vi "Handle Command.vi"(8 "error in":errorcluster, 10 "CMD in":refnum<class "Change Filter State CMD.lvclass">, 11 "Object In":refnum<class>) -> (0 "error out":errorcluster, 1 "Command Successful?":bool, 2 "CMD out":refnum<class "Change Filter State CMD.lvclass">, 3 "Object Out":refnum<class>)   [LabVIEW 2017, in "PAS Library.lvlib" / "Change Filter State CMD.lvclass"]
doc: "This VI will contain the code used to actually execute the request. If the request is successful, this will be indicated by the boolean output <b>Command Successful?</b>. The boolean output can then be used by the <b>Command Reply</b> which sends a reply if the reply queue is valid."
uses:
  Change Filter State CMD.lvclass
  Main/PAS.lvclass
  Change Filter State CMD.lvclass/Change Filter State CMD.ctl
  Cell/PAS Cell.lvclass/PAS Cell.ctl
  Cell/Write filter.vi
  Main/Read Cells.vi
  Main/Write Cells.vi
  Cell/PAS Cell.lvclass
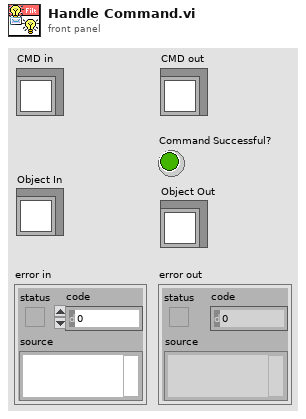
[diagram p1: front panel]
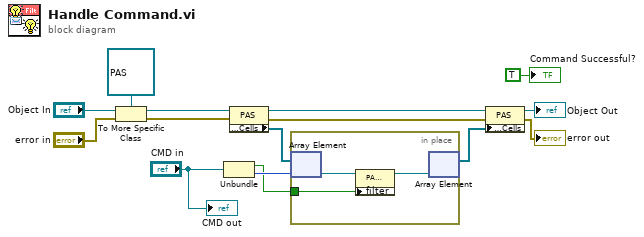
[diagram p0: block diagram]
diagram:
  n1 = To More Specific Class(target class=refnum<class "PAS.lvclass"> refnum ("PAS Library.lvlib:PAS"), reference="Object In", error in="error in") -> (specific class reference=w11:refnum<class "PAS.lvclass">, error out=w10:errorcluster)
  n2 = Unbundle("CMD in") -> (w7:bool, w8:u8)
  n3 = property class="PAS"(reference=w11, error in=w10) -> (reference out=w6:refnum<class "PAS.lvclass">, error out=w4:errorcluster, "Data Access:Cells"=w9:refnum<class "PAS Cell.lvclass">[])
  n4 = in-place {
    in-place-border: w7 -> [w17]
    n5 = in-place-array #1(w9, w8) -> (w18:refnum<class "PAS Cell.lvclass">)
    n6 = property class="PAS Cell"(reference=w18, "filter"=w17) -> (reference out=w16:refnum<class "PAS Cell.lvclass">)  [unwired: 1 in, 1 out]
    n7 = in-place-array #1(w16) -> (w5:refnum<class "PAS Cell.lvclass">[])  [unwired: 1 out]
  }
  n8 = property class="PAS"(reference=w6, error in=w4, "Data Access:Cells"=w5) -> (reference out=→"Object Out":refnum<class "PAS.lvclass">, error out=→"error out":errorcluster)
  "CMD out" <- "CMD in"
  "Command Successful?" <- TRUE ("Command Successful?")
